vi "[-50012] Front Panel is removed in Build Spec.vi"(8 "error in (no error)":errorcluster) -> (0 "error out":errorcluster)   [LabVIEW 2014, in "RefManager(dev).lvlib"]
uses:
  RefManager(dev).lvlib
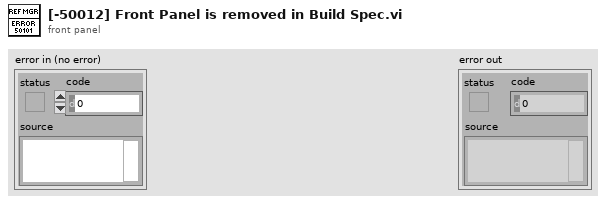
[diagram p1: front panel]
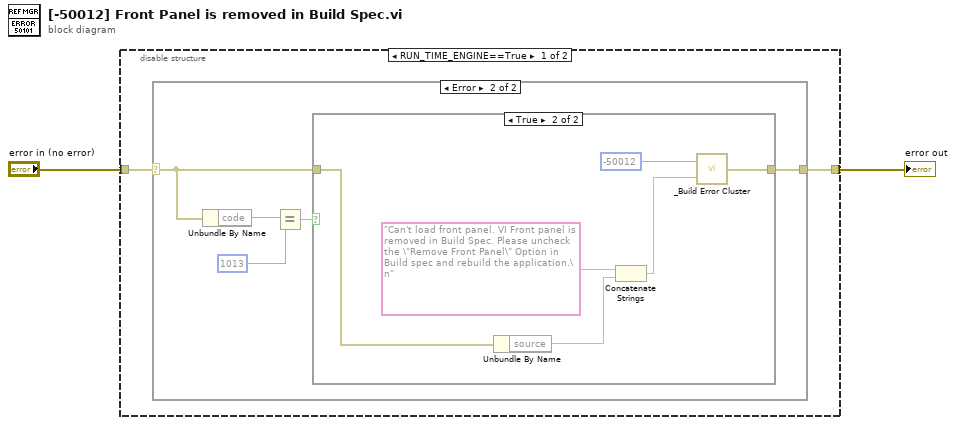
[diagram p0: block diagram]
diagram:
  n1 = disable-structure shown="RUN_TIME_ENGINE==True" {
    disable-tunnel: "error in (no error)" -> [w4 w18]
    disable-tunnel: [w3 w18] -> w1
    frame condition #0 {
      n2 = case shown="Error" w4 {
        selector: w4 -> [w5 w9]
        tunnel: [w5 w10] -> w3
        frame No Error {
        }
        frame Error {
          n3 = Unbundle By Name(w9) -> ("code"=w8:i32)
          n4 = Equal?(x=w8, y=1013) -> (x = y?=w6:bool)
          n5 = case shown="True" w6 {
            tunnel: [w11 w12] -> w10
            tunnel: w9 -> [w11 w16]
            frame False {
            }
            frame True {
              n6 = Unbundle By Name(w16) -> ("source"=w15:string)
              n7 = Concatenate Strings("Can't load front panel. VI Front panel is removed in Build Spec. Please uncheck the \"Remove Front Panel\" Option in Build spec and rebuild the application.\n" ("source"), w15) -> (w14:string)
              n8 = call <userlib>:"_Build Error Cluster.vi"("String to Prepend to source (\"\")"=w14, "code"=-50012) -> ("error out"=w12:errorcluster)
            }
          }
        }
      }
    }
    frame condition #1 (active) {
    }
  }
  "error out" <- w1
